vi "Create Temp Directory for Compile.vi"(8 "error in (no error)":errorcluster, 10 ".hhp file path":path, 11 "Help Path":path) -> (0 "error out":errorcluster, 2 "temp directory":path, 3 "temp .hhp path":path)   [LabVIEW 2015, in "HTML Help File Tools.lvlib"]
uses:
  HTML Help File Tools.lvlib
  Log FGV Operation Modes.ctl
  Error Location.ctl
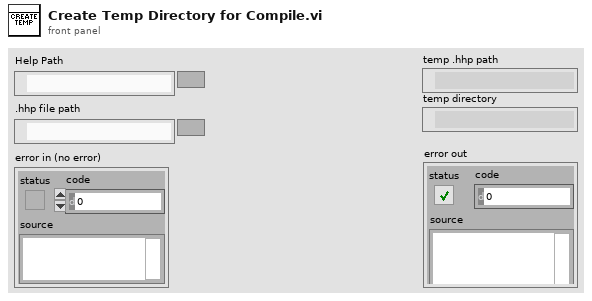
[diagram p1: front panel]
types:
  T1 = typedef "HTML Help File Tools.lvlib/Error Location.ctl" = enum16{"Delete tmp", "Compile HHP", "Find Install", "Create tmp", "Create HHP", "Find Help"}
  T2 = typedef "HTML Help File Tools.lvlib/Log FGV Operation Modes.ctl" = enum16{"Close", "Write", "Open File"}
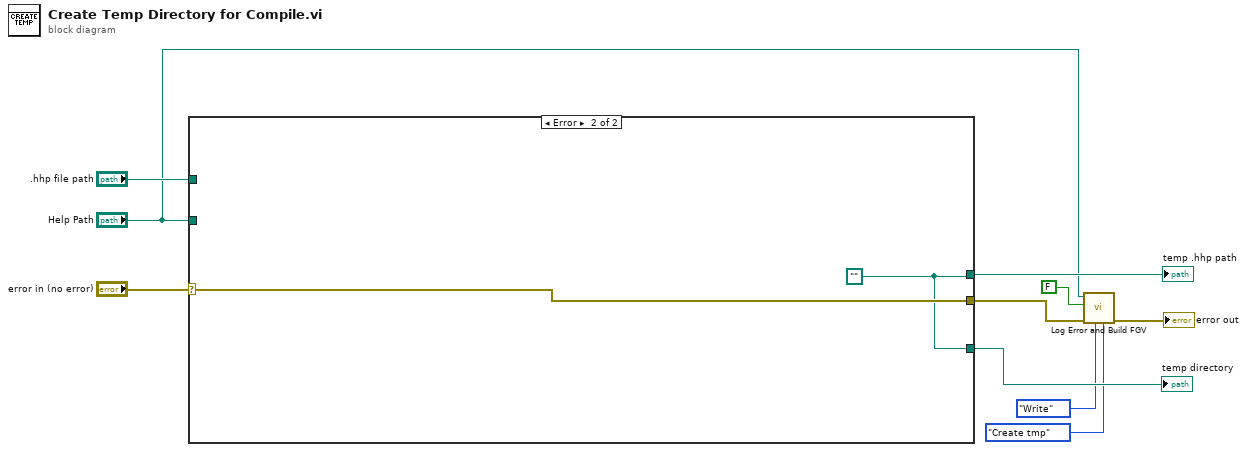
[diagram p0: block diagram]
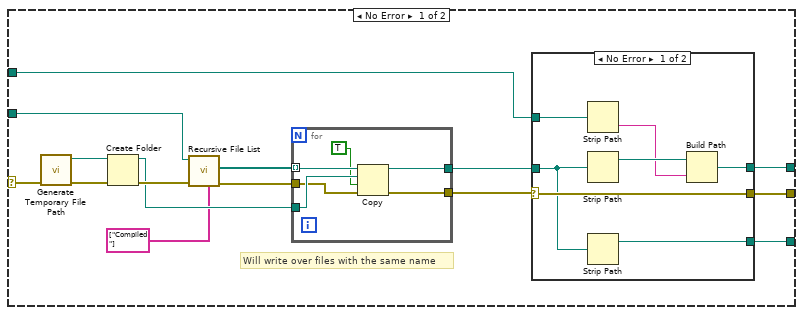
[diagram p2: hidden frame]
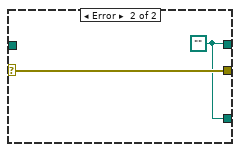
[diagram p3: hidden frame]
diagram:
  n1 = case shown="Error" "error in (no error)" {
    selector: "error in (no error)" -> [w19 w42]
    tunnel: "Help Path" -> [w18 _]
    tunnel: [w17 w42] -> w6
    tunnel: ".hhp file path" -> [w16 _]
    tunnel: [w15 w41] -> w8
    tunnel: [w13 w41] -> w7
    frame No Error {
      # "Will write over files with the same name"
      n2 = call <vilib>:"Generate Temporary File Path.vi"("error in (no error)"=w19) -> ("error out"=w25:errorcluster, "Unique Temporary File Path"=w24:path)  [unwired: 9 in]
      n3 = Create Folder(path (use dialog)=w24, error in=w25) -> (created path=w21:path, error out=w23:errorcluster)  [unwired: 1 in, 1 out]
      n4 = call <vilib>:"Recursive File List.vi"("Folders to Exclude"=string[] ["Compiled"], "error in (no error)"=w23, "Folder Path"=w18) -> ("error out"=w22:errorcluster, "All Files in Dir"=w11:path[])  [unwired: 4 in, 3 out]
      n5 = for {
        tunnel: w11 -> [w40] mode=indexing
        tunnel: w21 -> [w39]
        tunnel: w22 -> [w38]
        tunnel: [w37] -> w14
        tunnel: [w36] -> w20
        n6 = Copy(8:w38, 9:TRUE ("overwrite (F)"), 10:w39, 11:w40) -> (0:w36:errorcluster, 3:w37:path)  [unwired: 1 in, 1 out]
      }
      n7 = case shown="No Error" w20 {
        selector: w20 -> [w29 w34]
        tunnel: w14 -> [w27 _]
        tunnel: [w30 w33] -> w15
        tunnel: [w29 w34] -> w17
        tunnel: w16 -> [w28 _]
        tunnel: [w26 w33] -> w13
        frame No Error {
          n8 = Strip Path(path=w28) -> (name=w31:string)  [unwired: 1 out]
          n9 = Strip Path(path=w27) -> (stripped path=w32:path)  [unwired: 1 out]
          n10 = Strip Path(path=w27) -> (stripped path=w26:path)  [unwired: 1 out]
          n11 = Build Path(base path=w32, name or relative path=w31) -> (appended path=w30:path)
        }
        frame Error {
          w33 = path ""
        }
      }
    }
    frame Error {
      w41 = path ""
    }
  }
  "temp .hhp path" <- w8
  "temp directory" <- w7
  n12 = call "Log Error and Build FGV.vi"("Error Location"=Error_Location."Create tmp", "Operation Mode"=Log_FGV_Operation_Modes."Write", "error in"=w6, "Log Build Output?"=FALSE, "Help Documentation Path"="Help Path") -> ("error out"=→"error out":errorcluster)  [unwired: 6 in]
